vi "UpdateUserInterface.vi"(8 "error in (no error)":errorcluster, 10 "DataExchange":T1, 11 "StageController in":refnum<class "StageController.lvclass">) -> (0 "error out":errorcluster, 2 "DataExchange Out":T1, 3 "StageController out":refnum<class "StageController.lvclass">)   [LabVIEW 2020, in "StageController.lvlib" / "StageController.lvclass"]
uses:
  StageController.lvclass
  Model/Hardware Abstraction Layer/Component/Device/Device/DataExchange.ctl
  StageController.lvclass/StageController.ctl
  Model/Hardware Abstraction Layer/Component/GenericActor/GenericActor/GenericController.lvclass
  Interface/DataListener/DataListener.lvclass
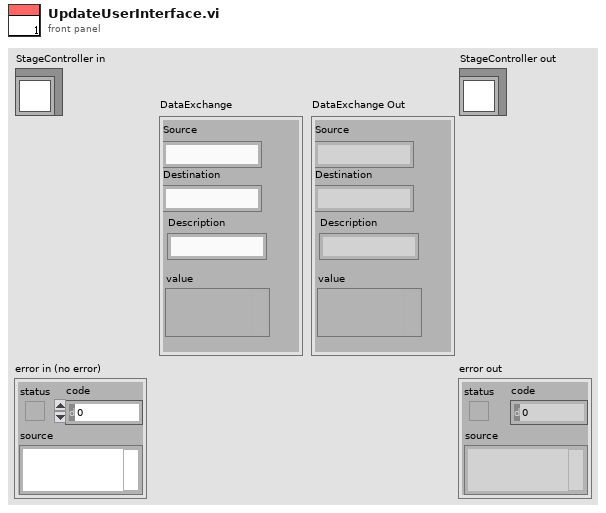
[diagram p1: front panel]
types:
  T1 = typedef "DataListener.lvclass/DataExchange.ctl" = cluster{"Source":string, "Destination":string, "Description":string, "value":variant}
  T2 = cluster{"Stage X Position":dbl, "Stage Y Position":dbl, "Stage Z Position":dbl}
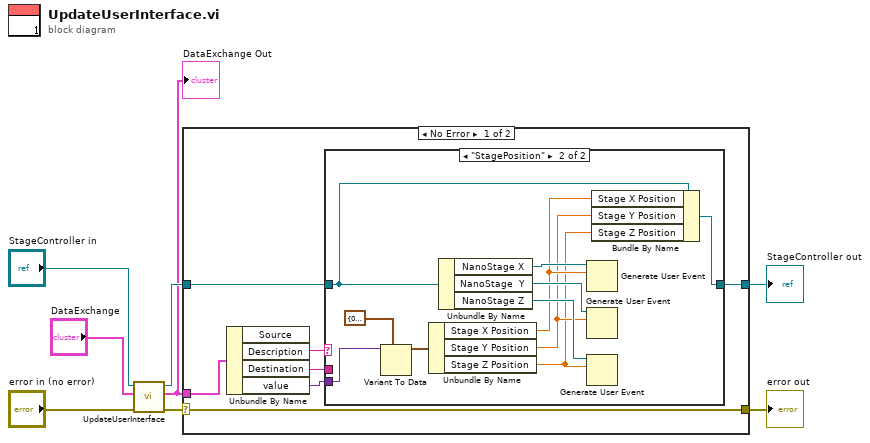
[diagram p0: block diagram]
diagram:
  n1 = call-parent "UpdateUserInterface.vi"("error in (no error)"="error in (no error)", "DataExchange"="DataExchange", "GenericController in"="StageController in") -> ("error out"=w4:errorcluster, "DataExchange Out"=w1:T1, "GenericController out"=w5:refnum<class "StageController.lvclass">)  [unwired: 6 in]
  "DataExchange Out" <- w1
  n2 = case shown="No Error" w4 {
    selector: w4 -> [w15 w29]
    tunnel: [w15 w29] -> w2
    tunnel: [w9 w28] -> w3
    tunnel: w5 -> [w10 w28]
    tunnel: w1 -> [w14 _]
    frame No Error {
      n3 = Unbundle By Name(w14) -> ("Description"=w11:string, "Destination"=w12:string, "value"=w13:variant)  [unwired: 1 out]
      n4 = case shown="\"StagePosition\"" w11 {
        tunnel: w13 -> [_ w27]
        tunnel: w12 -> [_ _]
        tunnel: w10 -> [w16 w21]
        tunnel: [w16 w20] -> w9
        frame Default {
        }
        frame "StagePosition" {
          n5 = Variant To Data(type=T2 {"Stage X Position"=0.0, "Stage Y Position"=0.0, "Stage Z Position"=0.0} ("Cluster"), Variant=w27) -> (data=w22:T2)  [unwired: 1 in, 1 out]
          n6 = Unbundle By Name(w22) -> ("Stage X Position"=w19:dbl, "Stage Y Position"=w18:dbl, "Stage Z Position"=w17:dbl)
          n7 = Unbundle By Name(w21) -> ("NanoStage X"=w26:refnum<user-event>, "NanoStage  Y"=w24:refnum<user-event>, "NanoStage Z"=w23:refnum<user-event>)
          n8 = Generate User Event(user event=w26, event data cluster=w19) -> ()  [unwired: 2 in, 2 out]
          n9 = Generate User Event(user event=w24, event data cluster=w18) -> ()  [unwired: 2 in, 2 out]
          n10 = Generate User Event(user event=w23, event data cluster=w17) -> ()  [unwired: 2 in, 2 out]
          n11 = Bundle By Name(cluster=w21, "Stage X Position"=w19, "Stage Y Position"=w18, "Stage Z Position"=w17) -> (w20:refnum<class "StageController.lvclass">)
        }
      }
    }
    frame Error {
    }
  }
  "error out" <- w2
  "StageController out" <- w3
